vi "h.ACQ.ScalePowerTraces.vi"(8 "X-axis":dbl[](array[numeric]), 9 "Offset":i32, 10 "Scale":u32, 11 "Spectrum":T1 {"Spectrum, db" format="%_8g"}) -> (2 "calibrated spectrum out":cluster{dbl[], dbl[]}, 3 "Spectrum, db":dbl[](array[numeric]))   [LabVIEW 2016, in "h.Library.lvlib"]
uses:
  h.Library.lvlib
  CTL/h.ACQ.Spectrum.ctl
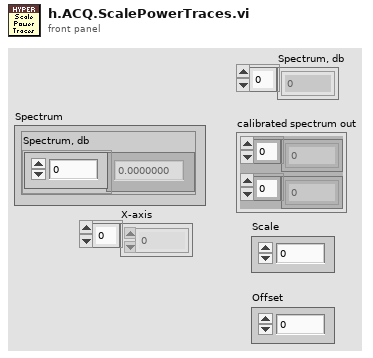
[diagram p1: front panel]
types:
  T1 = typedef "h.Library.lvlib/h.ACQ.Spectrum.ctl" = cluster{"Spectrum, db":dbl[]}
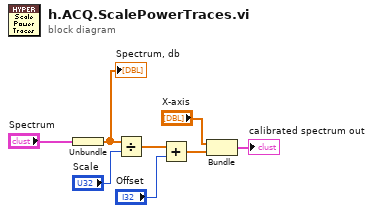
[diagram p0: block diagram]
diagram:
  n1 = Unbundle("Spectrum") -> ("Spectrum, db"=w8:dbl[])
  "Spectrum, db" <- w8
  n2 = Divide(x=w8, y="Scale") -> (x/y=w2:dbl[])
  n3 = Add(x=w2, y="Offset") -> (x+y=w4:dbl[])
  n4 = Bundle("X-axis"="X-axis", w4) -> (→"calibrated spectrum out":cluster{"X-axis":dbl[], dbl[]})  [unwired: 1 in]
